vi "CPCReadlior.vi"(10 "model":string, 11 "CPC port":refnum<visa-resource-name>) -> (2 "sigma part/cm3":dbl, 3 "concentration part/cm3":dbl)   [LabVIEW 2013]
panel:
  out "dup CPC port":refnum<visa-resource-name>
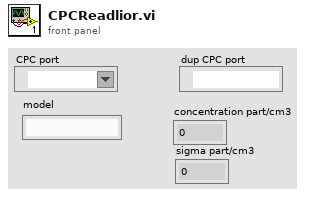
[diagram p1: front panel]
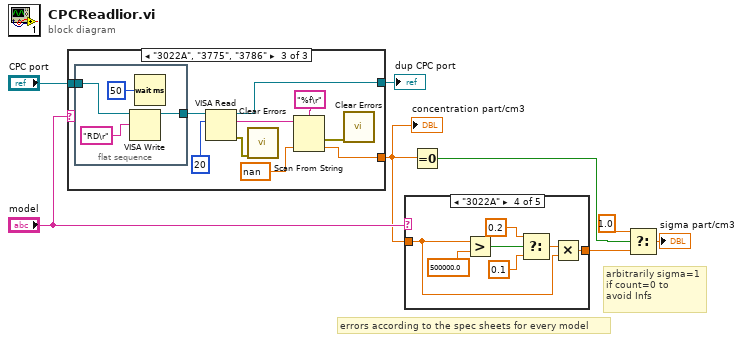
[diagram p0: block diagram]
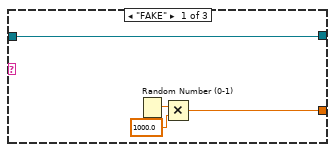
[diagram p2: hidden frame]
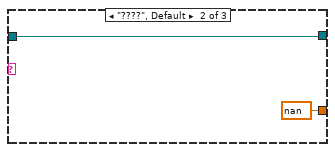
[diagram p3: hidden frame]
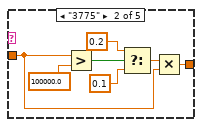
[diagram p5: hidden frame]
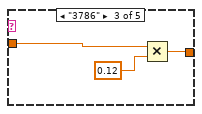
[diagram p6: hidden frame]
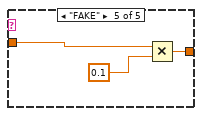
[diagram p7: hidden frame]
diagram:
  # "arbitrarily sigma=1\nif count=0 to\navoid Infs"
  # "errors according to the spec sheets for every model"
  n1 = case shown="\"3022A\", \"3775\", \"3786\"" "model" {
    tunnel: [w10 nan ("default value 1") w18] -> w4
    tunnel: "CPC port" -> [w9 w13 w17]
    tunnel: [w9 w13 w16] -> w6
    frame "FAKE" {
      n2 = Random Number (0-1)() -> (number: 0 to 1=w11:dbl)
      n3 = Multiply(x=w11, y=1000.0) -> (x*y=w10:dbl)
    }
    frame "????", Default {
    }
    frame "3022A", "3775", "3786" {
      n4 = flat-sequence {
        tunnel: [w28] -> w24
        tunnel: w17 -> [w26]
        frame #0 {
          n5 = VISA Write(VISA resource name=w26, write buffer="RD\r") -> (VISA resource name out=w28:refnum<visa-resource-name>)  [unwired: 1 in, 2 out]
          n6 = Wait (ms)(milliseconds to wait=u32 50) -> ()  [unwired: 1 out]
        }
      }
      n7 = VISA Read(VISA resource name=w24, byte count=u32 20) -> (VISA resource name out=w16:refnum<visa-resource-name>, read buffer=w22:string, error out=w19:errorcluster)  [unwired: 1 in, 1 out]
      n8 = call <vilib>:"Clear Errors.vi"("error in (no error)"=w19) -> ()  [unwired: 7 out]
      n9 = Scan From String(format string="%f\r", input string=w22, default 1=nan ("default value 1")) -> (error out=w20:errorcluster, output 1=w18:dbl)  [unwired: 2 in, 2 out]
      n10 = call <vilib>:"Clear Errors.vi"("error in (no error)"=w20) -> ()  [unwired: 7 out]
    }
  }
  "concentration part/cm3" <- w4
  "dup CPC port" <- w6
  n11 = case shown="\"3022A\"" "model" {
    tunnel: [w29 w30 w39 w40 w48] -> w5
    tunnel: w4 -> [w29 w31 w38 w41 w47]
    frame "????", Default {
    }
    frame "3775" {
      n12 = Greater?(x=w31, y=100000.0) -> (0:w33:bool)
      n13 = Select(t=0.2, s=w33, f=0.1) -> (s? t:f=w32:dbl)
      n14 = Multiply(x=w32, y=w31) -> (x*y=w30:dbl)
    }
    frame "3786" {
      n15 = Multiply(x=w38, y=0.12 ("x")) -> (x*y=w39:dbl)
    }
    frame "3022A" {
      n16 = Greater?(x=w41, y=500000.0) -> (0:w43:bool)
      n17 = Select(t=0.2, s=w43, f=0.1) -> (s? t:f=w42:dbl)
      n18 = Multiply(x=w42, y=w41) -> (x*y=w40:dbl)
    }
    frame "FAKE" {
      n19 = Multiply(x=w47, y=0.1 ("sigma part/cm3")) -> (x*y=w48:dbl)
    }
  }
  n20 = Equal To 0?(x=w4) -> (x = 0?=w2:bool)
  n21 = Select(t=1.0, s=w2, f=w5) -> (s? t:f=→"sigma part/cm3":dbl)
